vi "Linear_and_cumulative_Histogram(SubVI).vi"(8 "error in (no error)":errorcluster, 11 "Image GRAY":T2) -> (0 "error out":errorcluster, 2 "Linear Histogram":T1, 3 "Cumulative Histogram":u32[](array[numeric]))   [LabVIEW 2020]
uses:
  <vilib>/vision/Image Controls.llb/IMAQ Image.ctl
  <vilib>/vision/NI_Vision_Development_Module.lvlib
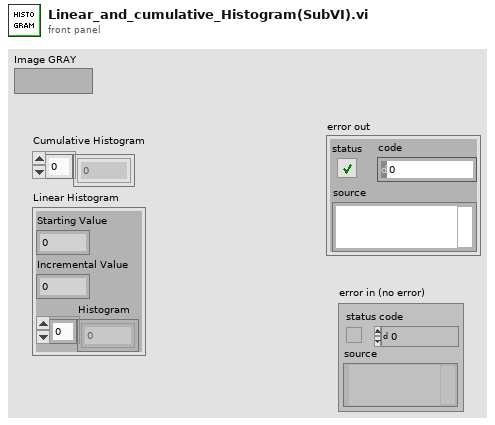
[diagram p1: front panel]
types:
  T1 = cluster{"Starting Value":sgl, "Incremental Value":sgl, "Histogram":u32[]}
  T2 = typedef "IMAQ Image.ctl" = refnum<image>
  T3 = cluster{"histogram":u32[], "Minimal Value":sgl, "Maximal Value":sgl, "Starting Value":sgl, "Interval Width":sgl, "Mean Value":sgl, "Standard  Variation":sgl, "Area (pixels)":i32}
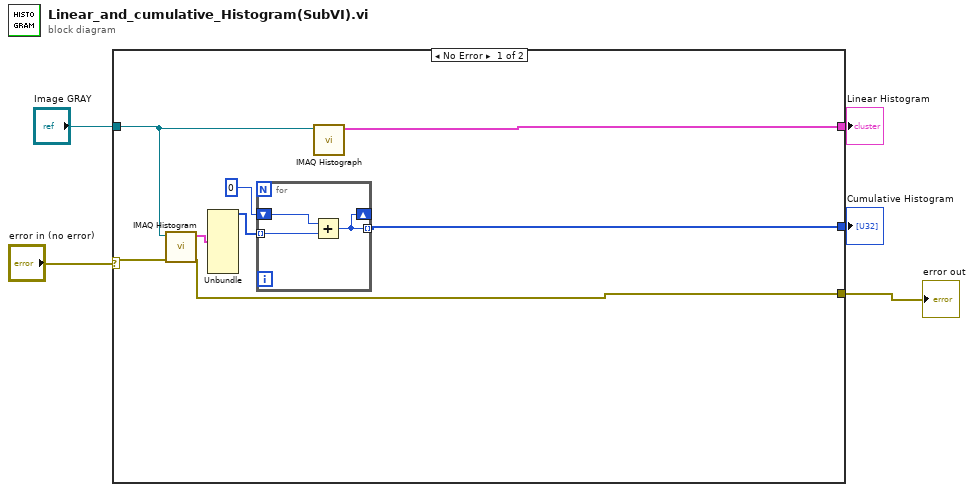
[diagram p0: block diagram]
diagram:
  n1 = case shown="No Error" "error in (no error)" {
    selector: "error in (no error)" -> [w7 w17]
    tunnel: "Image GRAY" -> [w8 _]
    tunnel: [w10 _] -> w4
    tunnel: [w9 _] -> w3
    tunnel: [w6 w17] -> w2
    frame No Error {
      n2 = call "IMAQ Histogram"("error in (no error)"=w7, "Image"=w8) -> ("error out"=w6:errorcluster, "Histogram Report"=w13:T3)  [unwired: 8 in]
      n3 = Unbundle(w13) -> ("histogram"=w11:u32[])  [unwired: 7 out]
      n4 = for {
        tunnel: w11 -> [w15] mode=indexing
        shift-right: [w14] -> _
        shift-left: u32 0 -> [w16]
        tunnel: [w14] -> w10 mode=indexing
        n5 = Add(x=w16, y=w15) -> (x+y=w14:u32)
      }
      n6 = call "IMAQ Histograph"("Image"=w8) -> ("Histogram Graph"=w9:T1)  [unwired: 7 in, 3 out]
    }
    frame Error {
    }
  }
  "Cumulative Histogram" <- w4
  "Linear Histogram" <- w3
  "error out" <- w2
